vi "Test for reachability.vi"(8 "error in (no error)":errorcluster, 10 "must be directly reachable?":bool, 11 "address":refnum<class "MacOS Network Address.lvclass">) -> (0 "error out":errorcluster, 2 "found?":bool, 3 "address out":refnum<class "Generic Network Address.lvclass">)   [LabVIEW 2020, in "NI_WFCN.lvlib" / "MacOS Network Address.lvclass"]
doc: "Determine whether the specified address is reachable."
uses:
  <vilib>/net/WFCN/Addressing/MacOS Network Address/MacOS Network Address.lvclass
  e:/builds/penguin/labview/branches/2020/dev/dist/vi.lib/net/WFCN/Addressing/Generic Network Address/Generic Network Address.lvclass
  <vilib>/net/WFCN/Addressing/Generic Network Address/Generic Network Address.lvclass
  <vilib>/net/WFCN/NI_WFCN.lvlib
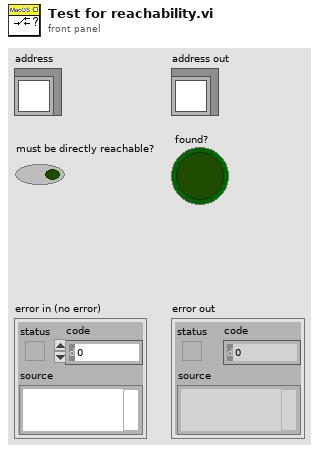
[diagram p1: front panel]
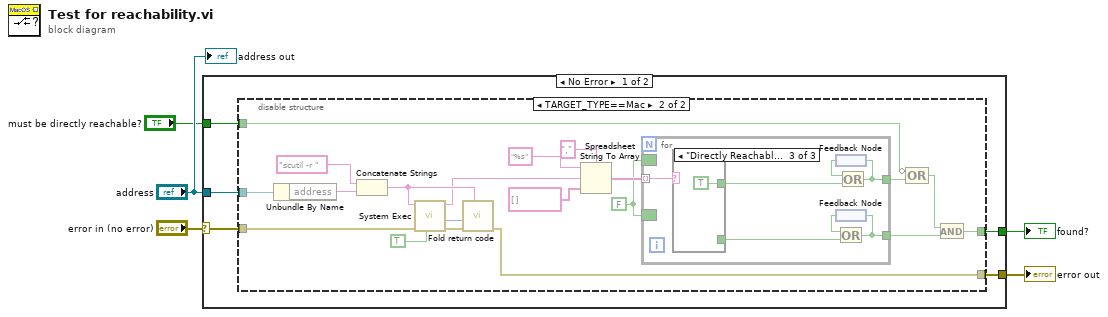
[diagram p0: block diagram]
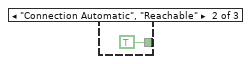
[diagram p4: hidden frame]
diagram:
  n1 = case shown="No Error" "error in (no error)" {
    selector: "error in (no error)" -> [w9 w40]
    tunnel: "address" -> [w10 _]
    tunnel: [w8 w40] -> w3
    tunnel: "must be directly reachable?" -> [w7 _]
    tunnel: [w6 _] -> w1
    frame No Error {
      n2 = disable-structure shown="TARGET_TYPE==Mac" {
        disable-tunnel: w10 -> [_ w30]
        disable-tunnel: w9 -> [_ w27]
        disable-tunnel: [_ w18] -> w8
        disable-tunnel: w7 -> [_ w12]
        disable-tunnel: [_ w11] -> w6
        frame condition #0 (active) {
        }
        frame condition #1 {
          w16 = FALSE
          n3 = Unbundle By Name(w30) -> ("address"=w28:string)
          n4 = Concatenate Strings("scutil -r ", w28) -> (w23:string)
          n5 = call <vilib>:"System Exec.vi"("run minimized? (F)"=TRUE, "error in (no error)"=w27, "command line"=w23) -> ("error out"=w25:errorcluster, "return code"=w24:i32, "standard output"=w17:string)  [unwired: 5 in, 1 out]
          n6 = call <vilib>:"Fold return code.vi"("command"=w23, "error in (no error)"=w25, "return code"=w24) -> ("error out"=w18:errorcluster)  [unwired: 8 in]
          n7 = Spreadsheet String To Array(delimiter (Tab)=",", format string="%s", spreadsheet string=w17, array type (2D Dbl)=string[] []) -> (array=w22:string[])
          n8 = for {
            tunnel: w22 -> [w37] mode=indexing
            border: w16 -> [_]
            border: w16 -> [_]
            tunnel: [w32] -> w13
            tunnel: [w31] -> w15
            n9 = case shown="\"Directly Reachable Address\"" w37 {
              tunnel: [_ TRUE _] -> w36
              tunnel: [_ _ TRUE] -> w34
              frame Default {
              }
              frame "Connection Automatic", "Reachable" {
              }
              frame "Directly Reachable Address" {
              }
            }
            n10 = feedback #1() -> (w33:bool)
            n11 = feedback #2() -> (w35:bool)
            n12 = Or(x=w35, y=w36) -> (x .or. y?=w31:bool)
            n13 = feedback-in #2(w31) -> ()
            n14 = Or(x=w33, y=w34) -> (x .or. y?=w32:bool)
            n15 = feedback-in #1(w32) -> ()
          }
          n16 = Compound Arithmetic op=OR(invert w12, w13) -> (w14:bool)
          n17 = And(x=w14, y=w15) -> (x .and. y?=w11:bool)
        }
      }
    }
    frame Error {
    }
  }
  "error out" <- w3
  "found?" <- w1
  "address out" <- "address"
